vi "convertRTPCOutputBytes.vi"(8 "FullScale":dbl=24576.0, 9 "SCCM":dbl=500.0, 10 "Active Instance":u8, 11 "Setpoint":dbl) -> (1 "Byte 2":u8, 2 "Byte 1":u8, 3 "Byte 0":u8)   [LabVIEW 2011]
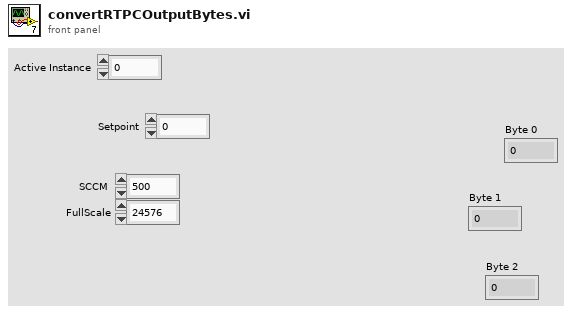
[diagram p1: front panel]
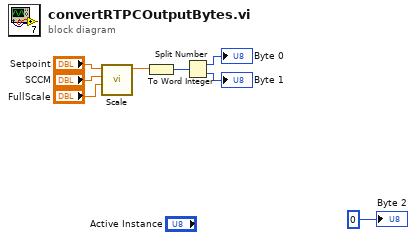
[diagram p0: block diagram]
diagram:
  n1 = call "Scale.vi"("Factor"="FullScale", "FullScale"="SCCM", "Input"="Setpoint") -> ("Output"=w7:dbl)  [unwired: 8 in]
  n2 = To Word Integer(number=w7) -> (16bit integer=w6:i16)
  n3 = Split Number(x=w6) -> (hi(x)=→"Byte 0":u8, lo(x)=→"Byte 1":u8)
  "Byte 2" <- u8 0 ("Byte 2")
